vi "Shutter-RT.vi"() -> ()   [LabVIEW 2016]
uses:
  Controls/Shutters.ctl
  Controls/Shutter Data.ctl
panel:
  in  "error in (no error)":errorcluster
  out "error out":errorcluster
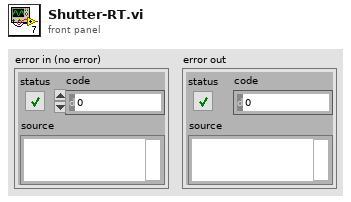
[diagram p1: front panel]
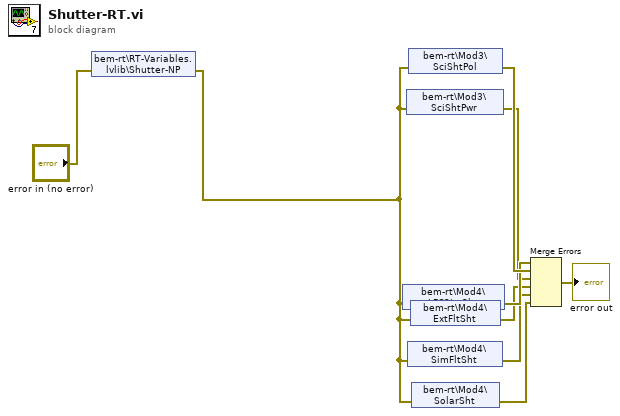
[diagram p0: block diagram]
diagram:
  n1 = shared-variable "bem-rt\\RT-Variables.lvlib\\Shutter-NP"(error in="error in (no error)") -> (error out=w1:errorcluster)  [unwired: 1 out]
  n2 = shared-variable "bem-rt\\Mod4\\LFCSimSht"(error in=w1) -> (error out=w7:errorcluster)  [unwired: 1 in]
  n3 = shared-variable "bem-rt\\Mod3\\SciShtPwr"(error in=w1) -> (error out=w6:errorcluster)  [unwired: 1 in]
  n4 = shared-variable "bem-rt\\Mod4\\SimFltSht"(error in=w1) -> (error out=w4:errorcluster)  [unwired: 1 in]
  n5 = shared-variable "bem-rt\\Mod3\\SciShtPol"(error in=w1) -> (error out=w8:errorcluster)  [unwired: 1 in]
  n6 = shared-variable "bem-rt\\Mod4\\ExtFltSht"(error in=w1) -> (error out=w5:errorcluster)  [unwired: 1 in]
  n7 = shared-variable "bem-rt\\Mod4\\SolarSht"(error in=w1) -> (error out=w3:errorcluster)  [unwired: 1 in]
  n8 = Merge Errors(w7, w8, w6, w5, w4, w3) -> (→"error out":errorcluster)
